vi "try.vi"() -> ()   [LabVIEW 2010]
panel:
  in  "CFG EDIT":string[][](table)
  out "Row Header Strings[]":string[](array[string])
  in  "Library function":string(tree)="sigDirMulStatInSet"
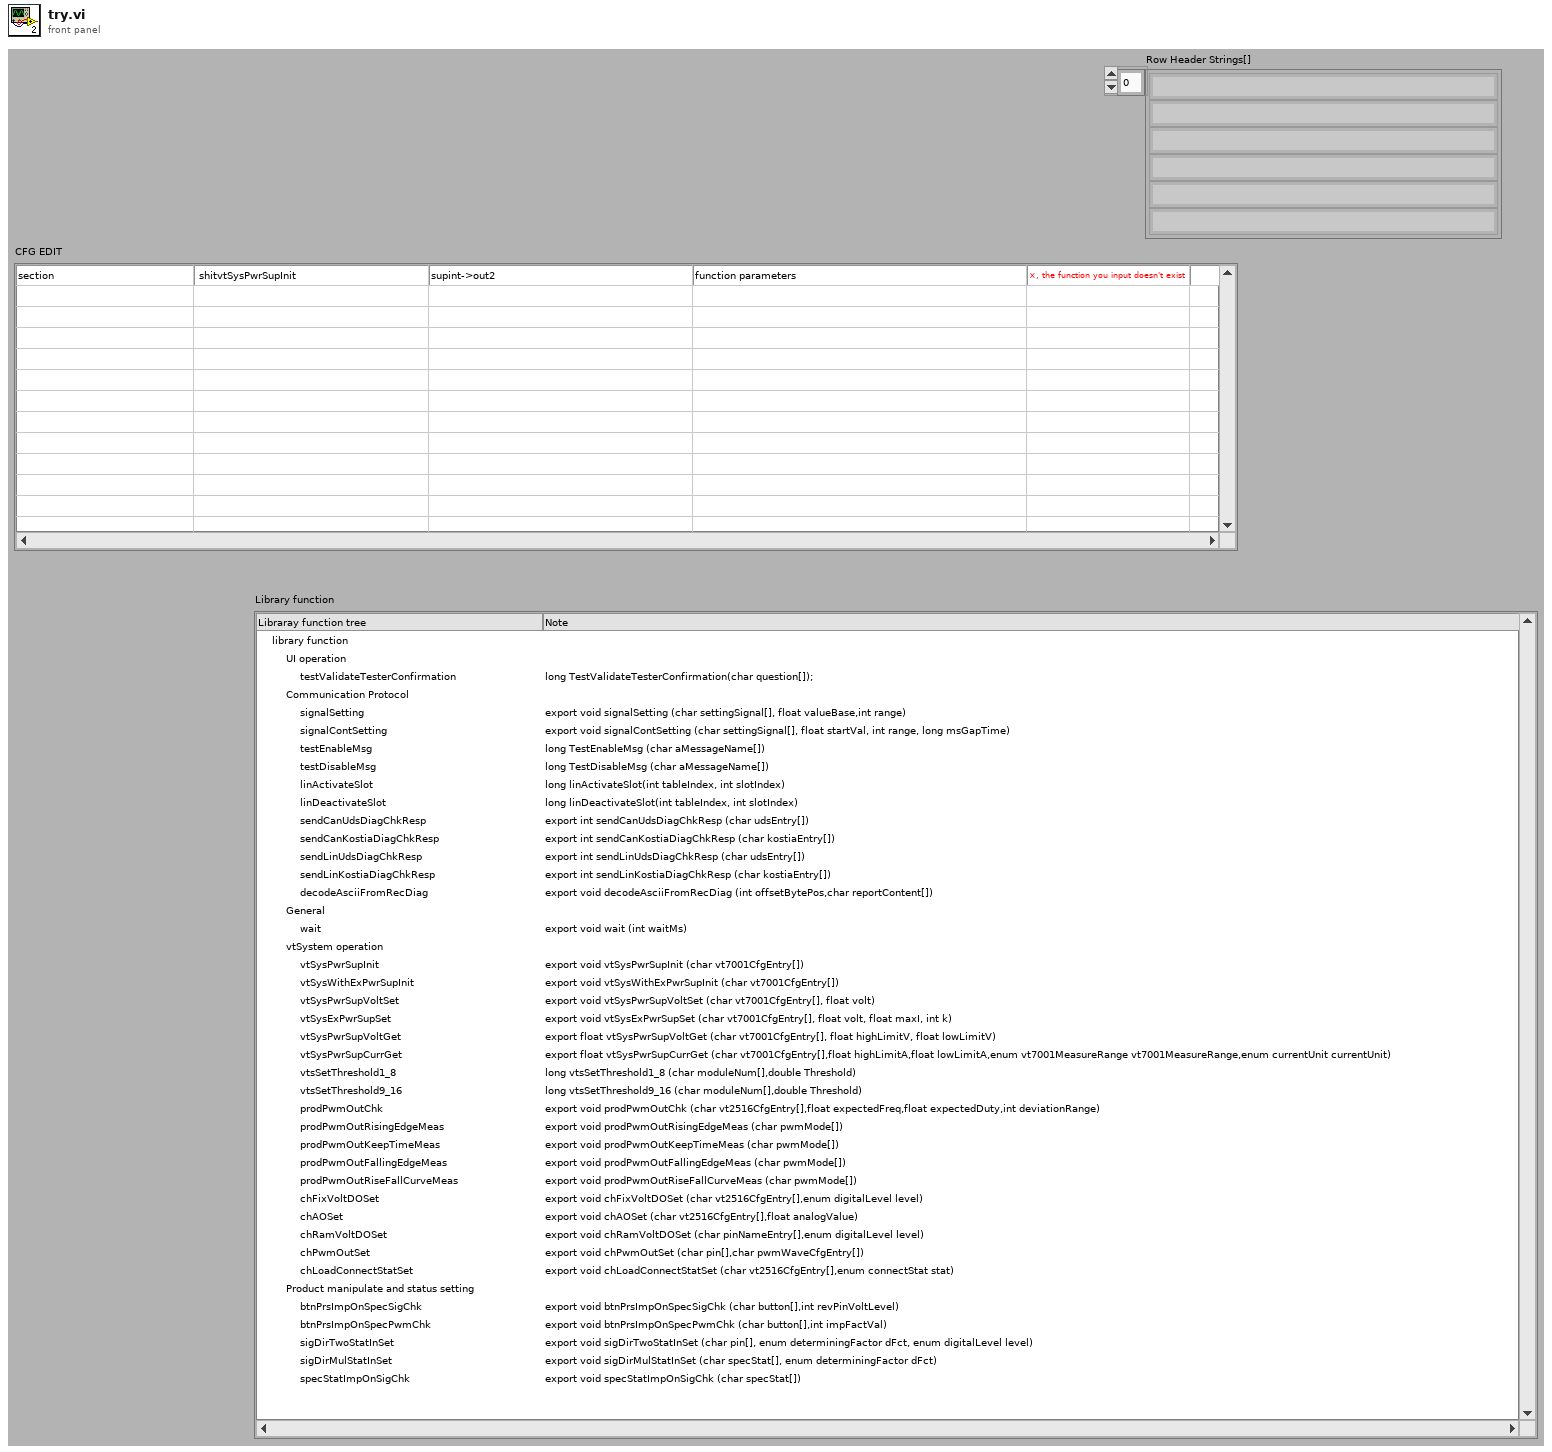
[diagram p1: front panel]
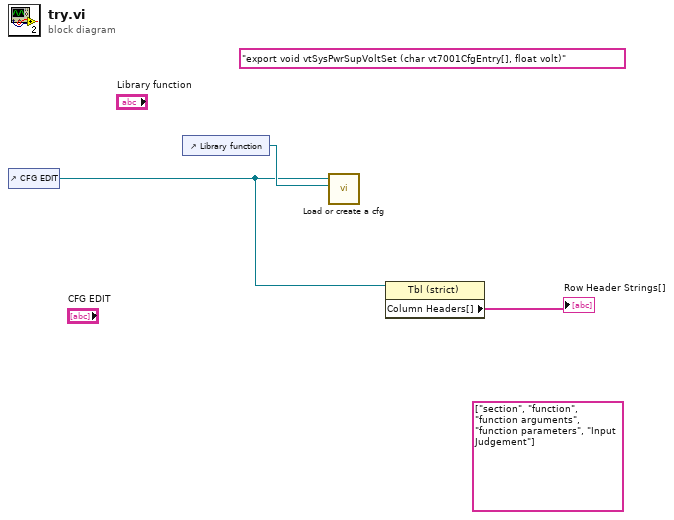
[diagram p0: block diagram]
diagram:
  (unwired) string[] ["section", "function", "function arguments", "function parameters", "Input Judgement"] ("Row Header Strings[]")
  (unwired) "export void vtSysPwrSupVoltSet (char vt7001CfgEntry[], float volt)"
  n1 = control-ref of="CFG EDIT"() -> (w1:refnum<vi>)
  n2 = control-ref of="Library function"() -> (w3:refnum<vi>)
  n3 = call "Load or create a cfg.vi"("Tree Refnum"=w3, "Tbl Refnum in"=w1) -> ()  [unwired: 6 in, 4 out]
  n4 = property class="Tbl (strict)"(reference=w1) -> ("Column Headers[]"=→"Row Header Strings[]":string[])  [unwired: 1 in, 2 out]
